vi "LockinDAQ.Read AI.vi"(8 "error in (no error)":errorcluster, 10 "AO []":waveform(dbl)[](array[waveform]), 11 "LockinDAQ":refnum<class "LockinDAQ.lvclass">=refnum) -> (0 "error out":errorcluster, 1 "AI time (ms)":u32=2, 2 "AI []":waveform(dbl)[](array[waveform]), 3 "LockinDAQ out":refnum<class "LockinDAQ.lvclass">)   [LabVIEW 2016, in "LockinDAQ.lvclass"]
uses:
  LockinDAQ.lvclass
  LockinDAQ.lvclass/LockinDAQ.ctl
  <vilib>/DAQmx/read.llb/DAQmx Read (Analog 1D Wfm NChan NSamp).vi
  <vilib>/DAQmx/miscellaneous.llb/DAQmx Fill In Error Info.vi
  <userlib>/_OpenG.lib/array/array.llb/Sort 1D Array (I32)__ogtk.vi
  <userlib>/_OpenG.lib/array/array.llb/Reorder 1D Array2 (Variant)__ogtk.vi
  <resource>/objmgr/daqmx.rc
panel:
  out "time to read samples":u32
  out "time to check for samples":u32
  out "Numeric":i32
  out "AvailSampPerChan 4":u32
  out "AvailSampPerChan 3":u32
  out "AvailSampPerChan 2":u32
  out "AvailSampPerChan 1":u32
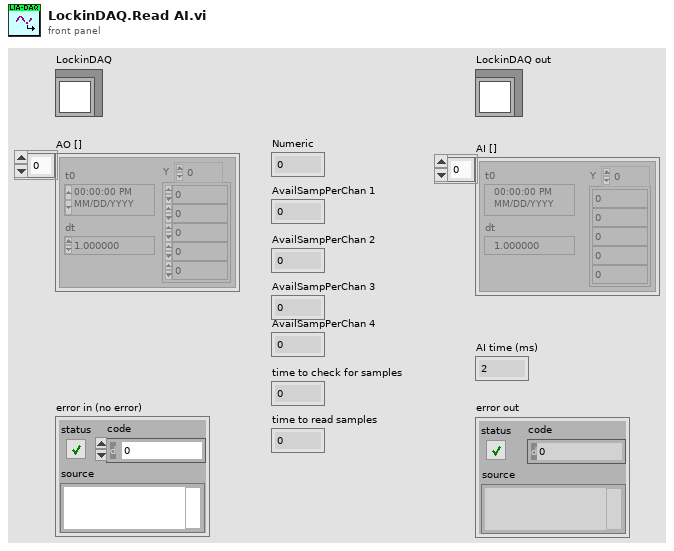
[diagram p1: front panel]
types:
  T1 = enum16{"static", "dynamic", "dynamic asynchronous"}
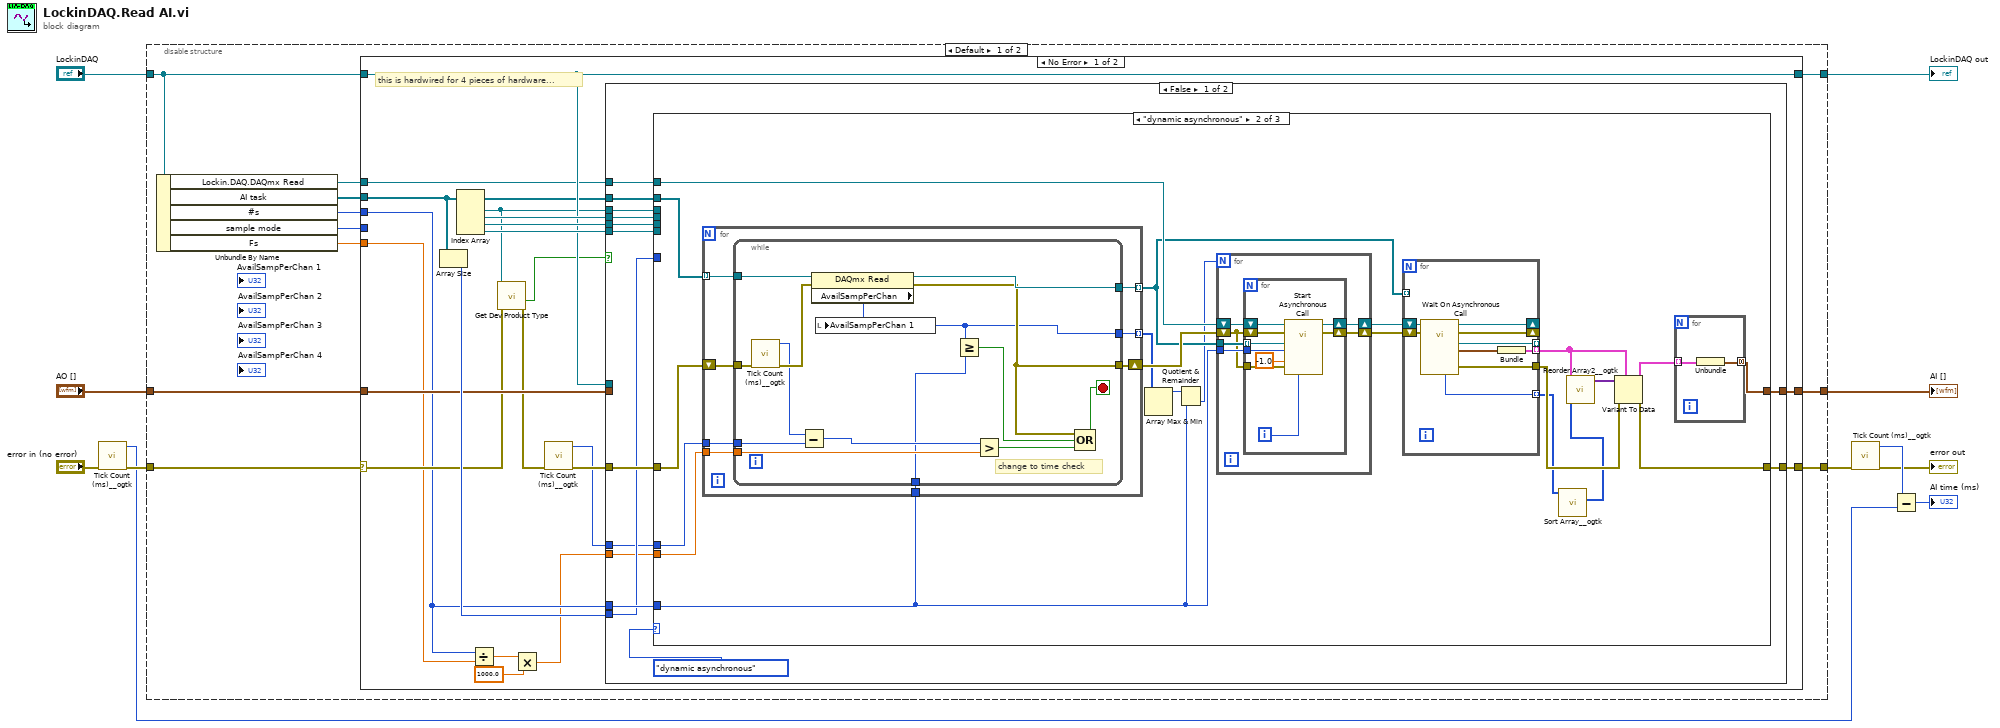
[diagram p0: block diagram]
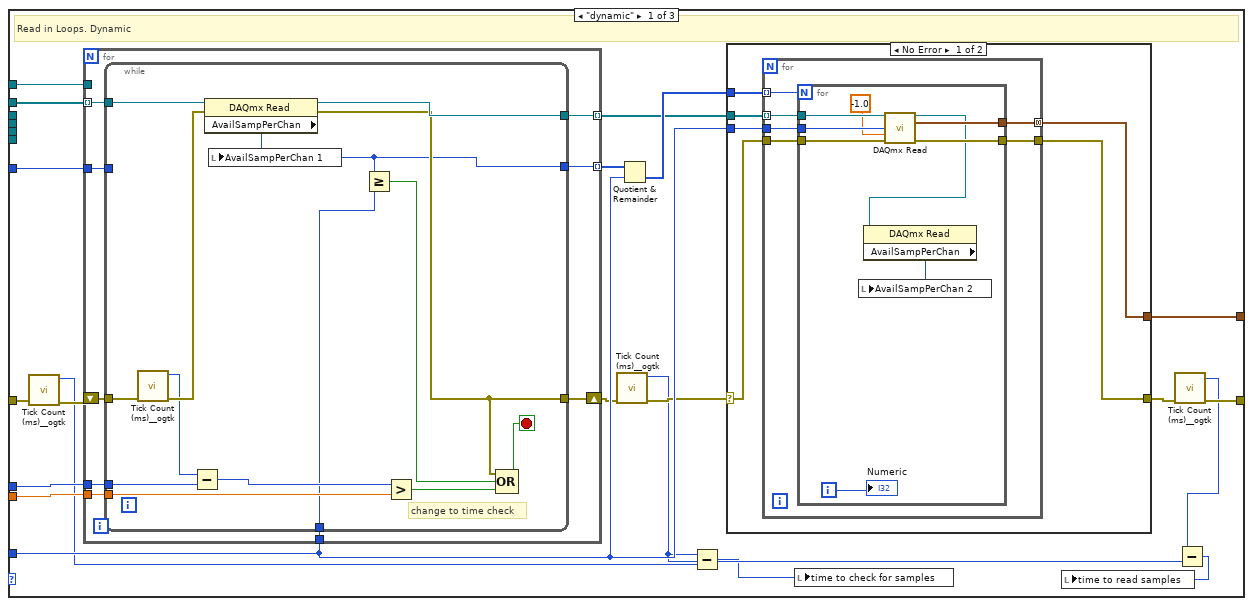
[diagram p2: hidden frame]
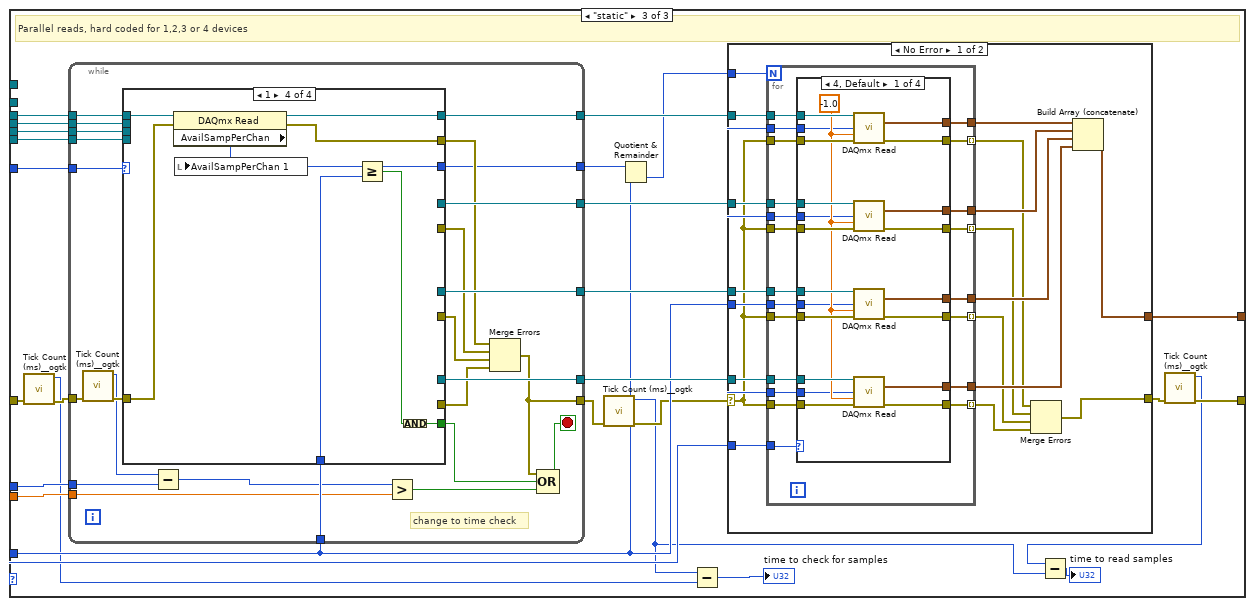
[diagram p4: hidden frame]
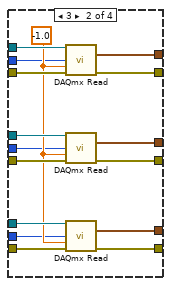
[diagram p5: hidden frame]
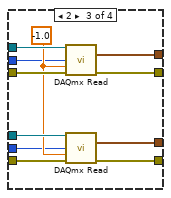
[diagram p6: hidden frame]
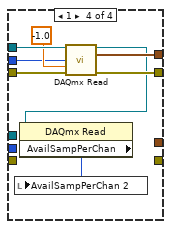
[diagram p7: hidden frame]
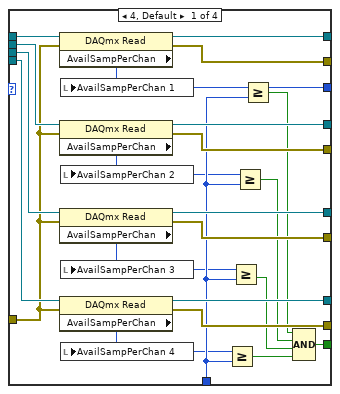
[diagram p9: hidden frame]
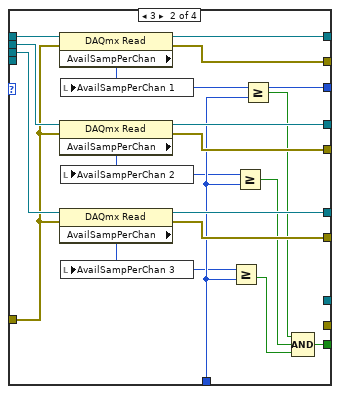
[diagram p10: hidden frame]
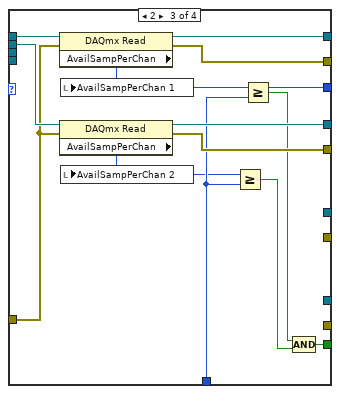
[diagram p11: hidden frame]
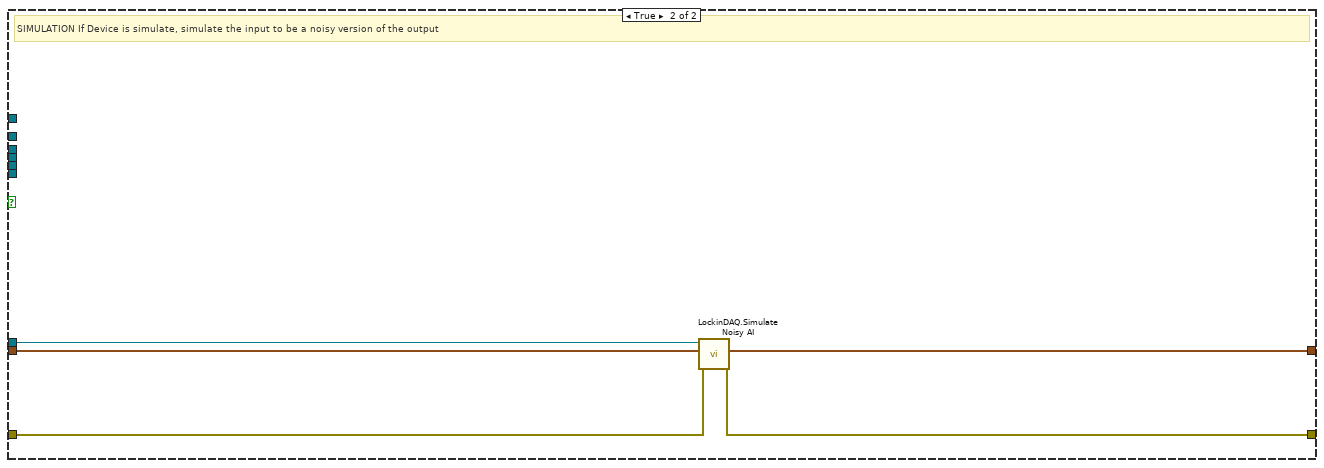
[diagram p12: hidden frame]
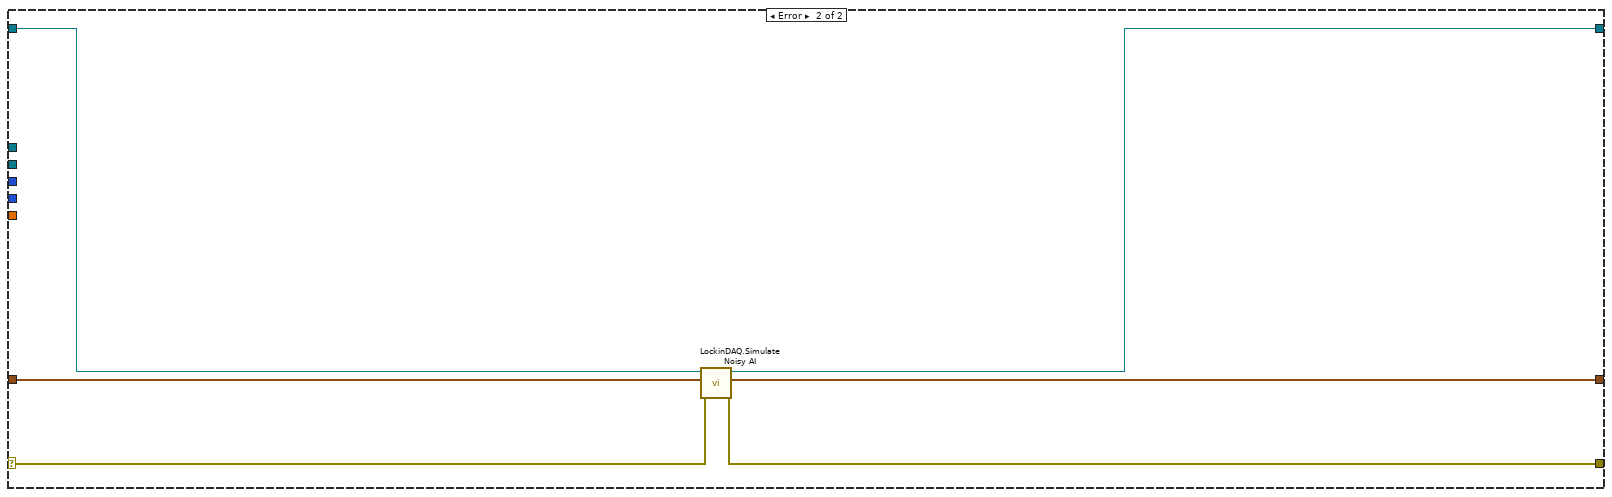
[diagram p13: hidden frame]
diagram:
  n1 = call <userlib>:"Tick Count (ms)__ogtk.vi"("error in (no error)"="error in (no error)") -> ("error out"=w8:errorcluster, "millisecond timer value"=w3:u32)  [unwired: 9 in]
  n2 = disable-structure shown="Default" {
    disable-tunnel: [w22 w413] -> w1
    disable-tunnel: [w19 w414] -> w7
    disable-tunnel: "LockinDAQ" -> [w17 _]
    disable-tunnel: "AO []" -> [w18 w413]
    disable-tunnel: w8 -> [w13 w414]
    disable-tunnel: [w16 _] -> w10
    frame condition #0 (active) {
      n3 = Unbundle By Name(w17) -> ("Lockin.DAQ.DAQmx Read"=w12:refnum<vi>, "AI task"=w15:refnum<k21>[], "#s"=w21:i32, "sample mode"=w20:i32, "Fs"=w14:dbl)
      n4 = case shown="No Error" w13 {
        selector: w13 -> [w33 w407]
        tunnel: [w43 w410] -> w22
        tunnel: w21 -> [w32 _]
        tunnel: w20 -> [_ _]
        tunnel: [w34 w409] -> w19
        tunnel: w18 -> [w38 w408]
        tunnel: w15 -> [w24 _]
        tunnel: w17 -> [w37 w412]
        tunnel: [w37 w411] -> w16
        tunnel: w14 -> [w31 _]
        tunnel: w12 -> [w23 _]
        frame No Error {
          # "this is hardwired for 4 pieces of hardware..."
          n5 = Array Size(array=w24) -> (size(s)=w39:i32)
          n6 = Index Array(array=w24) -> (element #1=w36:refnum<k21>, element #2=w40:refnum<k21>, element #3=w41:refnum<k21>, element #4=w42:refnum<k21>)  [unwired: 4 in]
          n7 = Divide(x=w32, y=w31) -> (x/y=w30:dbl)
          n8 = call "Get Dev Product Type.vi"("error in (no error)"=w33, "Refnum in"=w36) -> ("error out"=w27:errorcluster, "DevIsSimulated"=w35:bool)  [unwired: 6 in, 2 out]
          n9 = Multiply(x=w30, y=1000.0) -> (x*y=w26:dbl)
          n10 = call <userlib>:"Tick Count (ms)__ogtk.vi"("error in (no error)"=w27) -> ("error out"=w28:errorcluster, "millisecond timer value"=w25:u32)  [unwired: 9 in]
          n11 = case shown="False" w35 {
            tunnel: [w57 w402] -> w43
            tunnel: w42 -> [w56 _]
            tunnel: w41 -> [w55 _]
            tunnel: w40 -> [w54 _]
            tunnel: w36 -> [w53 _]
            tunnel: w32 -> [w52 _]
            tunnel: w28 -> [w50 w404]
            tunnel: w39 -> [w49 _]
            tunnel: [w51 w403] -> w34
            tunnel: w38 -> [_ w406]
            tunnel: w37 -> [_ w405]
            tunnel: w26 -> [w48 _]
            tunnel: w25 -> [w47 _]
            tunnel: w24 -> [w46 _]
            tunnel: w23 -> [w45 _]
            frame False {
              n12 = case shown="\"dynamic asynchronous\"" T1."dynamic asynchronous" ("Enum") {
                tunnel: [w78 w142 w218] -> w57
                tunnel: w56 -> [_ _ w217]
                tunnel: w55 -> [_ _ w216]
                tunnel: w54 -> [_ _ w215]
                tunnel: w53 -> [_ _ w214]
                tunnel: w52 -> [w77 w133 w209]
                tunnel: [w66 w126 w197] -> w51
                tunnel: w50 -> [w68 w139 w201]
                tunnel: w49 -> [w72 _ w208]
                tunnel: w48 -> [w76 w137 w207]
                tunnel: w47 -> [w73 w138 w204]
                tunnel: w46 -> [w71 w141 _]
                tunnel: w45 -> [w69 w136 _]
                frame "dynamic" {
                  # "Read in Loops. Dynamic"
                  n13 = call <userlib>:"Tick Count (ms)__ogtk.vi"("error in (no error)"=w68) -> ("error out"=w67:errorcluster, "millisecond timer value"=w62:u32)  [unwired: 9 in]
                  n14 = for {
                    tunnel: w77 -> [w87]
                    tunnel: w76 -> [w85]
                    tunnel: w72 -> [w81]
                    shift-right: [w83] -> w65
                    shift-left: w67 -> [w86]
                    tunnel: w71 -> [w80] mode=indexing
                    tunnel: w73 -> [w82]
                    tunnel: [w84] -> w74 mode=indexing
                    tunnel: [w79] -> w70 mode=indexing
                    tunnel: w69 -> [_]
                    n15 = while {
                      tunnel: [w101] -> w79
                      tunnel: w86 -> [w96]
                      tunnel: [w99] -> w83
                      tunnel: w87 -> [w88]
                      tunnel: w81 -> [_]
                      tunnel: w85 -> [w97]
                      tunnel: [w89] -> w84
                      tunnel: w82 -> [w93]
                      tunnel: w80 -> [w90]
                      stop <- w100 stop-if-true
                      # "change to time check"
                      n16 = call <userlib>:"Tick Count (ms)__ogtk.vi"("error in (no error)"=w96) -> ("error out"=w95:errorcluster, "millisecond timer value"=w94:u32)  [unwired: 9 in]
                      n17 = Subtract(x=w94, y=w93) -> (x-y=w92:u32)
                      n18 = property class="DAQmx Read"(reference=w90, error in=w95) -> (reference out=w101:refnum<k21>, error out=w99:errorcluster, "AvailSampPerChan"=w89:u32)
                      n19 = local write "AvailSampPerChan 1"(w89) -> ()
                      n20 = Greater Or Equal?(x=w89, y=w88) -> (x >= y?=w91:bool)
                      n21 = Greater?(x=w92, y=w97) -> (0:w98:bool)
                      n22 = Compound Arithmetic op=OR(w99, w91, w98) -> (w100:bool)
                    }
                  }
                  n23 = call <userlib>:"Tick Count (ms)__ogtk.vi"("error in (no error)"=w65) -> ("error out"=w64:errorcluster, "millisecond timer value"=w60:u32)  [unwired: 9 in]
                  n24 = Quotient & Remainder(x=w74, y=w77) -> (floor(x/y)=w75:u32[])  [unwired: 1 out]
                  n25 = Subtract(x=w60, y=w62) -> (x-y=w59:u32)
                  n26 = case shown="No Error" w64 {
                    selector: w64 -> [w104 w123]
                    tunnel: [w106 _] -> w78
                    tunnel: w77 -> [w107 _]
                    tunnel: [w103 w123] -> w63
                    tunnel: w75 -> [w105 _]
                    tunnel: w70 -> [w102 _]
                    frame No Error {
                      n27 = for {
                        tunnel: w107 -> [w113]
                        tunnel: [w112] -> w106 mode=concatenating
                        tunnel: w105 -> [w111] mode=indexing
                        tunnel: w104 -> [w110]
                        tunnel: [w109] -> w103
                        tunnel: w102 -> [w108] mode=indexing
                        n28 = for {
                          N: w111 -> [_]
                          tunnel: w108 -> [w122]
                          tunnel: w110 -> [w121]
                          tunnel: [w120] -> w112
                          tunnel: w113 -> [w119]
                          tunnel: [w118] -> w109
                          i -> [w117]
                          n29 = call-poly <vilib>:"DAQmx Read.vi"("task/channels in"=w122, "number of samples per channel"=w119, "timeout"=-1.0, "error in"=w121) -> ("task out"=w114:refnum<k21>, "data"=w120:waveform(dbl)[], "error out"=w118:errorcluster)  [unwired: 9 in]
                          n30 = property class="DAQmx Read"(reference=w114) -> ("AvailSampPerChan"=w115:u32)  [unwired: 1 in, 2 out]
                          n31 = local write "AvailSampPerChan 2"(w115) -> ()
                          "Numeric" <- w117
                        }
                      }
                    }
                    frame Error {
                    }
                  }
                  n32 = local write "time to check for samples"(w59) -> ()
                  n33 = call <userlib>:"Tick Count (ms)__ogtk.vi"("error in (no error)"=w63) -> ("error out"=w66:errorcluster, "millisecond timer value"=w61:u32)  [unwired: 9 in]
                  n34 = Subtract(x=w61, y=w60) -> (x-y=w58:u32)
                  n35 = local write "time to read samples"(w58) -> ()
                }
                frame "dynamic asynchronous" {
                  n36 = for {
                    tunnel: w133 -> [w167]
                    tunnel: w137 -> [w165]
                    shift-right: [w163] -> w140
                    shift-left: w139 -> [w166]
                    tunnel: w141 -> [w161] mode=indexing
                    tunnel: w138 -> [w162]
                    tunnel: [w164] -> w135 mode=indexing
                    tunnel: [w160] -> w132 mode=indexing
                    n37 = while {
                      tunnel: [w181] -> w160
                      tunnel: w166 -> [w176]
                      tunnel: [w179] -> w163
                      tunnel: w167 -> [w168]
                      tunnel: w165 -> [w177]
                      tunnel: [w169] -> w164
                      tunnel: w162 -> [w173]
                      tunnel: w161 -> [w170]
                      stop <- w180 stop-if-true
                      # "change to time check"
                      n38 = call <userlib>:"Tick Count (ms)__ogtk.vi"("error in (no error)"=w176) -> ("error out"=w175:errorcluster, "millisecond timer value"=w174:u32)  [unwired: 9 in]
                      n39 = Subtract(x=w174, y=w173) -> (x-y=w172:u32)
                      n40 = property class="DAQmx Read"(reference=w170, error in=w175) -> (reference out=w181:refnum<k21>, error out=w179:errorcluster, "AvailSampPerChan"=w169:u32)
                      n41 = local write "AvailSampPerChan 1"(w169) -> ()
                      n42 = Greater Or Equal?(x=w169, y=w168) -> (x >= y?=w171:bool)
                      n43 = Greater?(x=w172, y=w177) -> (0:w178:bool)
                      n44 = Compound Arithmetic op=OR(w179, w171, w178) -> (w180:bool)
                    }
                  }
                  n45 = Array Max & Min(array=w135) -> (max value=w134:u32)  [unwired: 3 out]
                  n46 = Quotient & Remainder(x=w134, y=w133) -> (floor(x/y)=w131:u32)  [unwired: 1 out]
                  n47 = for {
                    N: w131 -> [_]
                    tunnel: w132 -> [w148]
                    tunnel: w133 -> [w146]
                    shift-right: [w149] -> w143
                    shift-left: w140 -> [w145]
                    shift-right: [w150] -> w144
                    shift-left: w136 -> [w147]
                    n48 = for {
                      shift-right: [w159] -> w149
                      shift-left: w145 -> [w156]
                      shift-right: [w158] -> w150
                      shift-left: w147 -> [w157]
                      tunnel: w145 -> [w155]
                      tunnel: w148 -> [w154] mode=indexing
                      tunnel: w146 -> [w152]
                      i -> [w151]
                      n49 = call-by-ref "Start Asynchronous Call"(reference=w157, error in=w156, "Refnum in"=w154, "number of samples per channel"=w152, "timeout"=-1.0, 11:"error in (no error)"=w155, "ID in"=w151) -> (reference out=w158:refnum<vi>, error out=w159:errorcluster)  [unwired: 7 in, 4 out]
                    }
                  }
                  n50 = for {
                    shift-right: [w189] -> _
                    shift-left: w143 -> [w191]
                    shift-right: [w190] -> _
                    shift-left: w144 -> [w192]
                    tunnel: [w186] -> _ mode=indexing
                    tunnel: [w188] -> w127
                    tunnel: [w185] -> w129 mode=indexing
                    tunnel: [w184] -> w125 mode=indexing
                    tunnel: w132 -> [_] mode=indexing
                    n51 = call-by-ref "Wait On Asynchronous Call"(reference=w192, error in=w191) -> (reference out=w190:refnum<vi>, error out=w189:errorcluster, "Refnum out"=w186:refnum<k21>, "data"=w187:waveform(dbl)[], "ID out"=w184:i32, 15:"error out"=w188:errorcluster)  [unwired: 12 in]
                    n52 = Bundle("data"=w187) -> (w185:cluster{"data":waveform(dbl)[]})  [unwired: 1 in]
                  }
                  n53 = call-poly <userlib>:"Sort Array__ogtk.vi"("Array in"=w125) -> ("Sorted Pointers"=w124:i32[])  [unwired: 9 in, 1 out]
                  n54 = call-poly <userlib>:"Reorder Array2__ogtk.vi"("indices"=w124, "array"=w129) -> ("reordered array"=w130:variant[])  [unwired: 9 in]
                  n55 = Variant To Data(error in=w127, type=w129, Variant=w130) -> (data=w128:cluster{"data":waveform(dbl)[]}[], error out=w126:errorcluster)
                  n56 = for {
                    tunnel: [w183] -> w142 mode=concatenating
                    tunnel: w128 -> [w182] mode=indexing
                    n57 = Unbundle(w182) -> ("data"=w183:waveform(dbl)[])
                  }
                }
                frame "static" {
                  # "Parallel reads, hard coded for 1,2,3 or 4 devices"
                  n58 = call <userlib>:"Tick Count (ms)__ogtk.vi"("error in (no error)"=w201) -> ("error out"=w200:errorcluster, "millisecond timer value"=w199:u32)  [unwired: 9 in]
                  n59 = while {
                    tunnel: w217 -> [w339]
                    tunnel: w216 -> [w338]
                    tunnel: w215 -> [w337]
                    tunnel: w214 -> [w336]
                    tunnel: [w335] -> w213
                    tunnel: [w334] -> w212
                    tunnel: [w333] -> w211
                    tunnel: [w332] -> w210
                    tunnel: w200 -> [w319]
                    tunnel: [w321] -> w203
                    tunnel: w209 -> [w331]
                    tunnel: w208 -> [w330]
                    tunnel: w207 -> [w323]
                    tunnel: [w320] -> w205
                    tunnel: w204 -> [w316]
                    stop <- w329 stop-if-true
                    # "change to time check"
                    n60 = call <userlib>:"Tick Count (ms)__ogtk.vi"("error in (no error)"=w319) -> ("error out"=w318:errorcluster, "millisecond timer value"=w317:u32)  [unwired: 9 in]
                    n61 = case shown="1" w330 {
                      tunnel: w339 -> [w362 _ _ _]
                      tunnel: w338 -> [w361 w380 _ _]
                      tunnel: w337 -> [w360 w379 w393 _]
                      tunnel: w336 -> [w359 w378 w392 w401]
                      tunnel: [w358 w377 w391 w400] -> w335
                      tunnel: [w357 w376 w390 _] -> w334
                      tunnel: [w356 w375 _ _] -> w333
                      tunnel: [w355 _ _ _] -> w332
                      tunnel: [w354 w374 w389 w399] -> w325
                      tunnel: [w353 w373 w388 _] -> w326
                      tunnel: [w352 w372 _ _] -> w327
                      tunnel: [w351 _ _ _] -> w328
                      tunnel: w318 -> [w350 w371 w387 w398]
                      tunnel: w331 -> [w345 w367 w384 w396]
                      tunnel: [w341 w364 w382 w395] -> w322
                      tunnel: [w340 w363 w381 w394] -> w320
                      frame 4, Default {
                        n62 = property class="DAQmx Read"(reference=w359, error in=w350) -> (reference out=w358:refnum<k21>, error out=w354:errorcluster, "AvailSampPerChan"=w340:u32)
                        n63 = property class="DAQmx Read"(reference=w360, error in=w350) -> (reference out=w357:refnum<k21>, error out=w353:errorcluster, "AvailSampPerChan"=w342:u32)
                        n64 = property class="DAQmx Read"(reference=w361, error in=w350) -> (reference out=w356:refnum<k21>, error out=w352:errorcluster, "AvailSampPerChan"=w343:u32)
                        n65 = property class="DAQmx Read"(reference=w362, error in=w350) -> (reference out=w355:refnum<k21>, error out=w351:errorcluster, "AvailSampPerChan"=w344:u32)
                        n66 = local write "AvailSampPerChan 1"(w340) -> ()
                        n67 = local write "AvailSampPerChan 2"(w342) -> ()
                        n68 = local write "AvailSampPerChan 3"(w343) -> ()
                        n69 = local write "AvailSampPerChan 4"(w344) -> ()
                        n70 = Greater Or Equal?(x=w344, y=w345) -> (x >= y?=w349:bool)
                        n71 = Greater Or Equal?(x=w343, y=w345) -> (x >= y?=w348:bool)
                        n72 = Greater Or Equal?(x=w342, y=w345) -> (x >= y?=w347:bool)
                        n73 = Greater Or Equal?(x=w340, y=w345) -> (x >= y?=w346:bool)
                        n74 = Compound Arithmetic op=AND(w346, w347, w348, w349) -> (w341:bool)
                      }
                      frame 3 {
                        n75 = property class="DAQmx Read"(reference=w378, error in=w371) -> (reference out=w377:refnum<k21>, error out=w374:errorcluster, "AvailSampPerChan"=w363:u32)
                        n76 = property class="DAQmx Read"(reference=w379, error in=w371) -> (reference out=w376:refnum<k21>, error out=w373:errorcluster, "AvailSampPerChan"=w365:u32)
                        n77 = property class="DAQmx Read"(reference=w380, error in=w371) -> (reference out=w375:refnum<k21>, error out=w372:errorcluster, "AvailSampPerChan"=w366:u32)
                        n78 = local write "AvailSampPerChan 1"(w363) -> ()
                        n79 = local write "AvailSampPerChan 2"(w365) -> ()
                        n80 = local write "AvailSampPerChan 3"(w366) -> ()
                        n81 = Greater Or Equal?(x=w366, y=w367) -> (x >= y?=w370:bool)
                        n82 = Greater Or Equal?(x=w365, y=w367) -> (x >= y?=w369:bool)
                        n83 = Greater Or Equal?(x=w363, y=w367) -> (x >= y?=w368:bool)
                        n84 = Compound Arithmetic op=AND(w368, w369, w370) -> (w364:bool)
                      }
                      frame 2 {
                        n85 = property class="DAQmx Read"(reference=w392, error in=w387) -> (reference out=w391:refnum<k21>, error out=w389:errorcluster, "AvailSampPerChan"=w381:u32)
                        n86 = property class="DAQmx Read"(reference=w393, error in=w387) -> (reference out=w390:refnum<k21>, error out=w388:errorcluster, "AvailSampPerChan"=w383:u32)
                        n87 = local write "AvailSampPerChan 1"(w381) -> ()
                        n88 = local write "AvailSampPerChan 2"(w383) -> ()
                        n89 = Greater Or Equal?(x=w383, y=w384) -> (x >= y?=w386:bool)
                        n90 = Greater Or Equal?(x=w381, y=w384) -> (x >= y?=w385:bool)
                        n91 = Compound Arithmetic op=AND(w385, w386) -> (w382:bool)
                      }
                      frame 1 {
                        n92 = property class="DAQmx Read"(reference=w401, error in=w398) -> (reference out=w400:refnum<k21>, error out=w399:errorcluster, "AvailSampPerChan"=w394:u32)
                        n93 = local write "AvailSampPerChan 1"(w394) -> ()
                        n94 = Greater Or Equal?(x=w394, y=w396) -> (x >= y?=w397:bool)
                        n95 = Compound Arithmetic op=AND(w397) -> (w395:bool)
                      }
                    }
                    n96 = Subtract(x=w317, y=w316) -> (x-y=w315:u32)
                    n97 = Greater?(x=w315, y=w323) -> (0:w324:bool)
                    n98 = Merge Errors(w325, w326, w327, w328) -> (w321:errorcluster)
                    n99 = Compound Arithmetic op=OR(w321, w322, w324) -> (w329:bool)
                  }
                  n100 = call <userlib>:"Tick Count (ms)__ogtk.vi"("error in (no error)"=w203) -> ("error out"=w202:errorcluster, "millisecond timer value"=w194:u32)  [unwired: 9 in]
                  n101 = Quotient & Remainder(x=w205, y=w209) -> (floor(x/y)=w206:u32)  [unwired: 1 out]
                  n102 = Subtract(x=w194, y=w199) -> (x-y=→"time to check for samples":u32)
                  n103 = case shown="No Error" w202 {
                    selector: w202 -> [w219 w314]
                    tunnel: [w236 _] -> w218
                    tunnel: w213 -> [w235 _]
                    tunnel: w212 -> [w234 _]
                    tunnel: w211 -> [w233 _]
                    tunnel: w210 -> [w232 _]
                    tunnel: w209 -> [w228 _]
                    tunnel: [w223 w314] -> w198
                    tunnel: w208 -> [w221 _]
                    tunnel: w206 -> [w220 _]
                    frame No Error {
                      n104 = for {
                        N: w220 -> [_]
                        tunnel: w235 -> [w257]
                        tunnel: w234 -> [w256]
                        tunnel: w233 -> [w255]
                        tunnel: w232 -> [w254]
                        tunnel: w219 -> [w253]
                        tunnel: w219 -> [w252]
                        tunnel: w219 -> [w251]
                        tunnel: w219 -> [w250]
                        tunnel: [w249] -> w231
                        tunnel: [w248] -> w222
                        tunnel: [w247] -> w230
                        tunnel: [w246] -> w229
                        tunnel: w228 -> [w245]
                        tunnel: w228 -> [w244]
                        tunnel: w228 -> [w243]
                        tunnel: w228 -> [w242]
                        tunnel: [w241] -> w227 mode=indexing
                        tunnel: [w240] -> w226 mode=indexing
                        tunnel: [w239] -> w225 mode=indexing
                        tunnel: [w238] -> w224 mode=indexing
                        tunnel: w221 -> [w237]
                        n105 = case shown="4, Default" w237 {
                          tunnel: w257 -> [w278 w294 w305 w313]
                          tunnel: w256 -> [w277 w293 w304 _]
                          tunnel: w255 -> [w276 w292 _ _]
                          tunnel: w254 -> [w275 _ _ _]
                          tunnel: w253 -> [w274 w291 w303 w312]
                          tunnel: w252 -> [w273 w290 w302 _]
                          tunnel: w251 -> [w272 w289 _ _]
                          tunnel: w250 -> [w271 _ _ _]
                          tunnel: [w269 w287 w300 _] -> w249
                          tunnel: [w268 w286 w299 w310] -> w248
                          tunnel: [w267 w285 _ _] -> w247
                          tunnel: [w266 _ _ _] -> w246
                          tunnel: w245 -> [w265 _ _ _]
                          tunnel: w244 -> [w264 w284 w298 w309]
                          tunnel: w243 -> [w263 w283 _ _]
                          tunnel: w242 -> [w262 w282 w297 _]
                          tunnel: [w261 w281 w296 w308] -> w241
                          tunnel: [w260 w280 w295 _] -> w240
                          tunnel: [w259 w279 _ _] -> w239
                          tunnel: [w258 _ _ _] -> w238
                          frame 4, Default {
                            w270 = -1.0 ("timeout")
                            n106 = call-poly <vilib>:"DAQmx Read.vi"("task/channels in"=w278, "number of samples per channel"=w264, "timeout"=w270, "error in"=w274) -> ("data"=w268:waveform(dbl)[], "error out"=w261:errorcluster)  [unwired: 9 in, 1 out]
                            n107 = call-poly <vilib>:"DAQmx Read.vi"("task/channels in"=w277, "number of samples per channel"=w262, "timeout"=w270, "error in"=w273) -> ("data"=w269:waveform(dbl)[], "error out"=w260:errorcluster)  [unwired: 9 in, 1 out]
                            n108 = call-poly <vilib>:"DAQmx Read.vi"("task/channels in"=w276, "number of samples per channel"=w263, "timeout"=w270, "error in"=w272) -> ("data"=w267:waveform(dbl)[], "error out"=w259:errorcluster)  [unwired: 9 in, 1 out]
                            n109 = call-poly <vilib>:"DAQmx Read.vi"("task/channels in"=w275, "number of samples per channel"=w265, "timeout"=w270, "error in"=w271) -> ("data"=w266:waveform(dbl)[], "error out"=w258:errorcluster)  [unwired: 9 in, 1 out]
                          }
                          frame 3 {
                            w288 = -1.0 ("timeout")
                            n110 = call-poly <vilib>:"DAQmx Read.vi"("task/channels in"=w294, "number of samples per channel"=w284, "timeout"=w288, "error in"=w291) -> ("data"=w286:waveform(dbl)[], "error out"=w281:errorcluster)  [unwired: 9 in, 1 out]
                            n111 = call-poly <vilib>:"DAQmx Read.vi"("task/channels in"=w293, "number of samples per channel"=w282, "timeout"=w288, "error in"=w290) -> ("data"=w287:waveform(dbl)[], "error out"=w280:errorcluster)  [unwired: 9 in, 1 out]
                            n112 = call-poly <vilib>:"DAQmx Read.vi"("task/channels in"=w292, "number of samples per channel"=w283, "timeout"=w288, "error in"=w289) -> ("data"=w285:waveform(dbl)[], "error out"=w279:errorcluster)  [unwired: 9 in, 1 out]
                          }
                          frame 2 {
                            w301 = -1.0 ("timeout")
                            n113 = call-poly <vilib>:"DAQmx Read.vi"("task/channels in"=w305, "number of samples per channel"=w298, "timeout"=w301, "error in"=w303) -> ("data"=w299:waveform(dbl)[], "error out"=w296:errorcluster)  [unwired: 9 in, 1 out]
                            n114 = call-poly <vilib>:"DAQmx Read.vi"("task/channels in"=w304, "number of samples per channel"=w297, "timeout"=w301, "error in"=w302) -> ("data"=w300:waveform(dbl)[], "error out"=w295:errorcluster)  [unwired: 9 in, 1 out]
                          }
                          frame 1 {
                            n115 = call-poly <vilib>:"DAQmx Read.vi"("task/channels in"=w313, "number of samples per channel"=w309, "timeout"=-1.0, "error in"=w312) -> ("task out"=w306:refnum<k21>, "data"=w310:waveform(dbl)[], "error out"=w308:errorcluster)  [unwired: 9 in]
                            n116 = property class="DAQmx Read"(reference=w306) -> ("AvailSampPerChan"=w307:u32)  [unwired: 1 in, 2 out]
                            n117 = local write "AvailSampPerChan 2"(w307) -> ()
                          }
                        }
                      }
                      n118 = Merge Errors(w227, w226, w225, w224) -> (w223:errorcluster)
                      n119 = Build Array (concatenate)(w222, w231, w230, w229) -> (w236:waveform(dbl)[])
                    }
                    frame Error {
                    }
                  }
                  n120 = call <userlib>:"Tick Count (ms)__ogtk.vi"("error in (no error)"=w198) -> ("error out"=w197:errorcluster, "millisecond timer value"=w196:u32)  [unwired: 9 in]
                  n121 = Subtract(x=w196, y=w194) -> (x-y=→"time to read samples":u32)
                }
              }
            }
            frame True {
              # "SIMULATION If Device is simulate, simulate the input to be a noisy version of the output"
              n122 = call "LockinDAQ.Simulate Noisy AI.vi"("error in (no error)"=w404, "AI []"=w406, "LockinDAQ"=w405) -> ("error out"=w403:errorcluster, "Noisy AI []"=w402:waveform(dbl)[])  [unwired: 6 in, 1 out]
            }
          }
        }
        frame Error {
          n123 = call "LockinDAQ.Simulate Noisy AI.vi"("error in (no error)"=w407, "AI []"=w408, "LockinDAQ"=w412) -> ("error out"=w409:errorcluster, "Noisy AI []"=w410:waveform(dbl)[], "LockinDAQ out"=w411:refnum<class "LockinDAQ.lvclass">)  [unwired: 6 in]
        }
      }
    }
    frame condition #1 {
    }
  }
  "AI []" <- w1
  "LockinDAQ out" <- w10
  n124 = call <userlib>:"Tick Count (ms)__ogtk.vi"("error in (no error)"=w7) -> ("error out"=→"error out":errorcluster, "millisecond timer value"=w6:u32)  [unwired: 9 in]
  n125 = Subtract(x=w6, y=w3) -> (x-y=→"AI time (ms)":u32)
